vi "fitting modified.vi"(0 "fitting type":i8(ring), 5 "2D data":dbl[][](array[numeric]), 9 "force guess?":bool, 11 "intial guess value":dbl[](array[numeric])) -> (3 "number of function calls":i32 caption="函数调用次数", 6 "best fit":dbl[][](array[numeric]), 10 "best fit parameters":dbl[](array[numeric]))   [LabVIEW 2013]
uses:
  <vilib>/gmath/NumericalOptimization/Nonlinear Curve Fit LM.vi
  <vilib>/gmath/NI_Gmath.lvlib
panel:
  out "initial value 3":dbl[](array[numeric])
  out "sub3":dbl[][](array[numeric])
  out "split 2":dbl
  out "split 1":dbl
  in  "initial value 2":dbl[](array[numeric])
  in  "initial value 1":dbl[](array[numeric])
  in  "sub2":dbl[][](array[numeric])
  in  "sub1":dbl[][](array[numeric])
  in  "yc":dbl[](array[numeric])
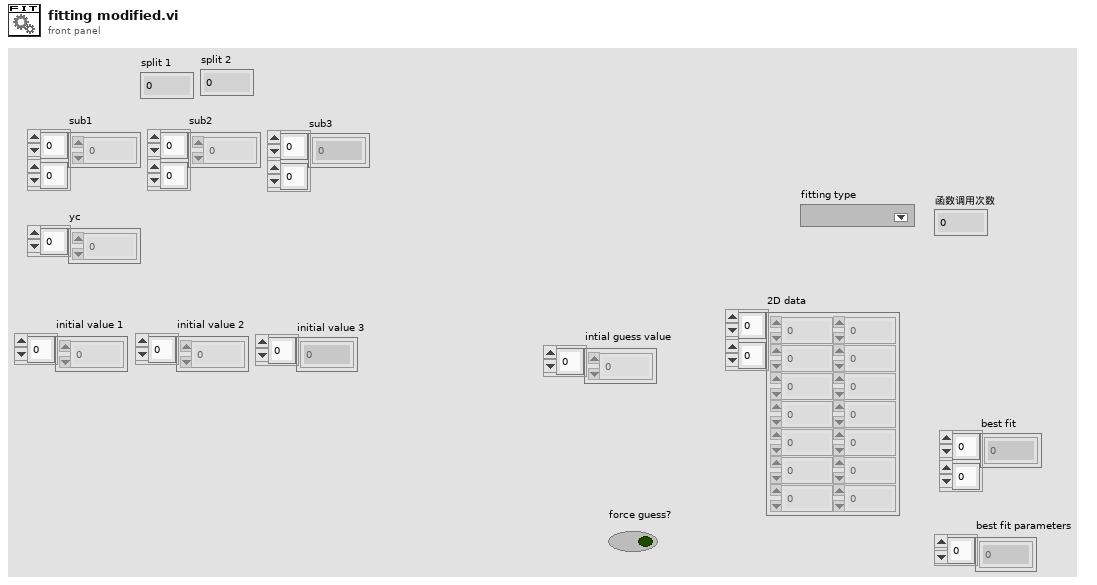
[diagram p1: front panel]
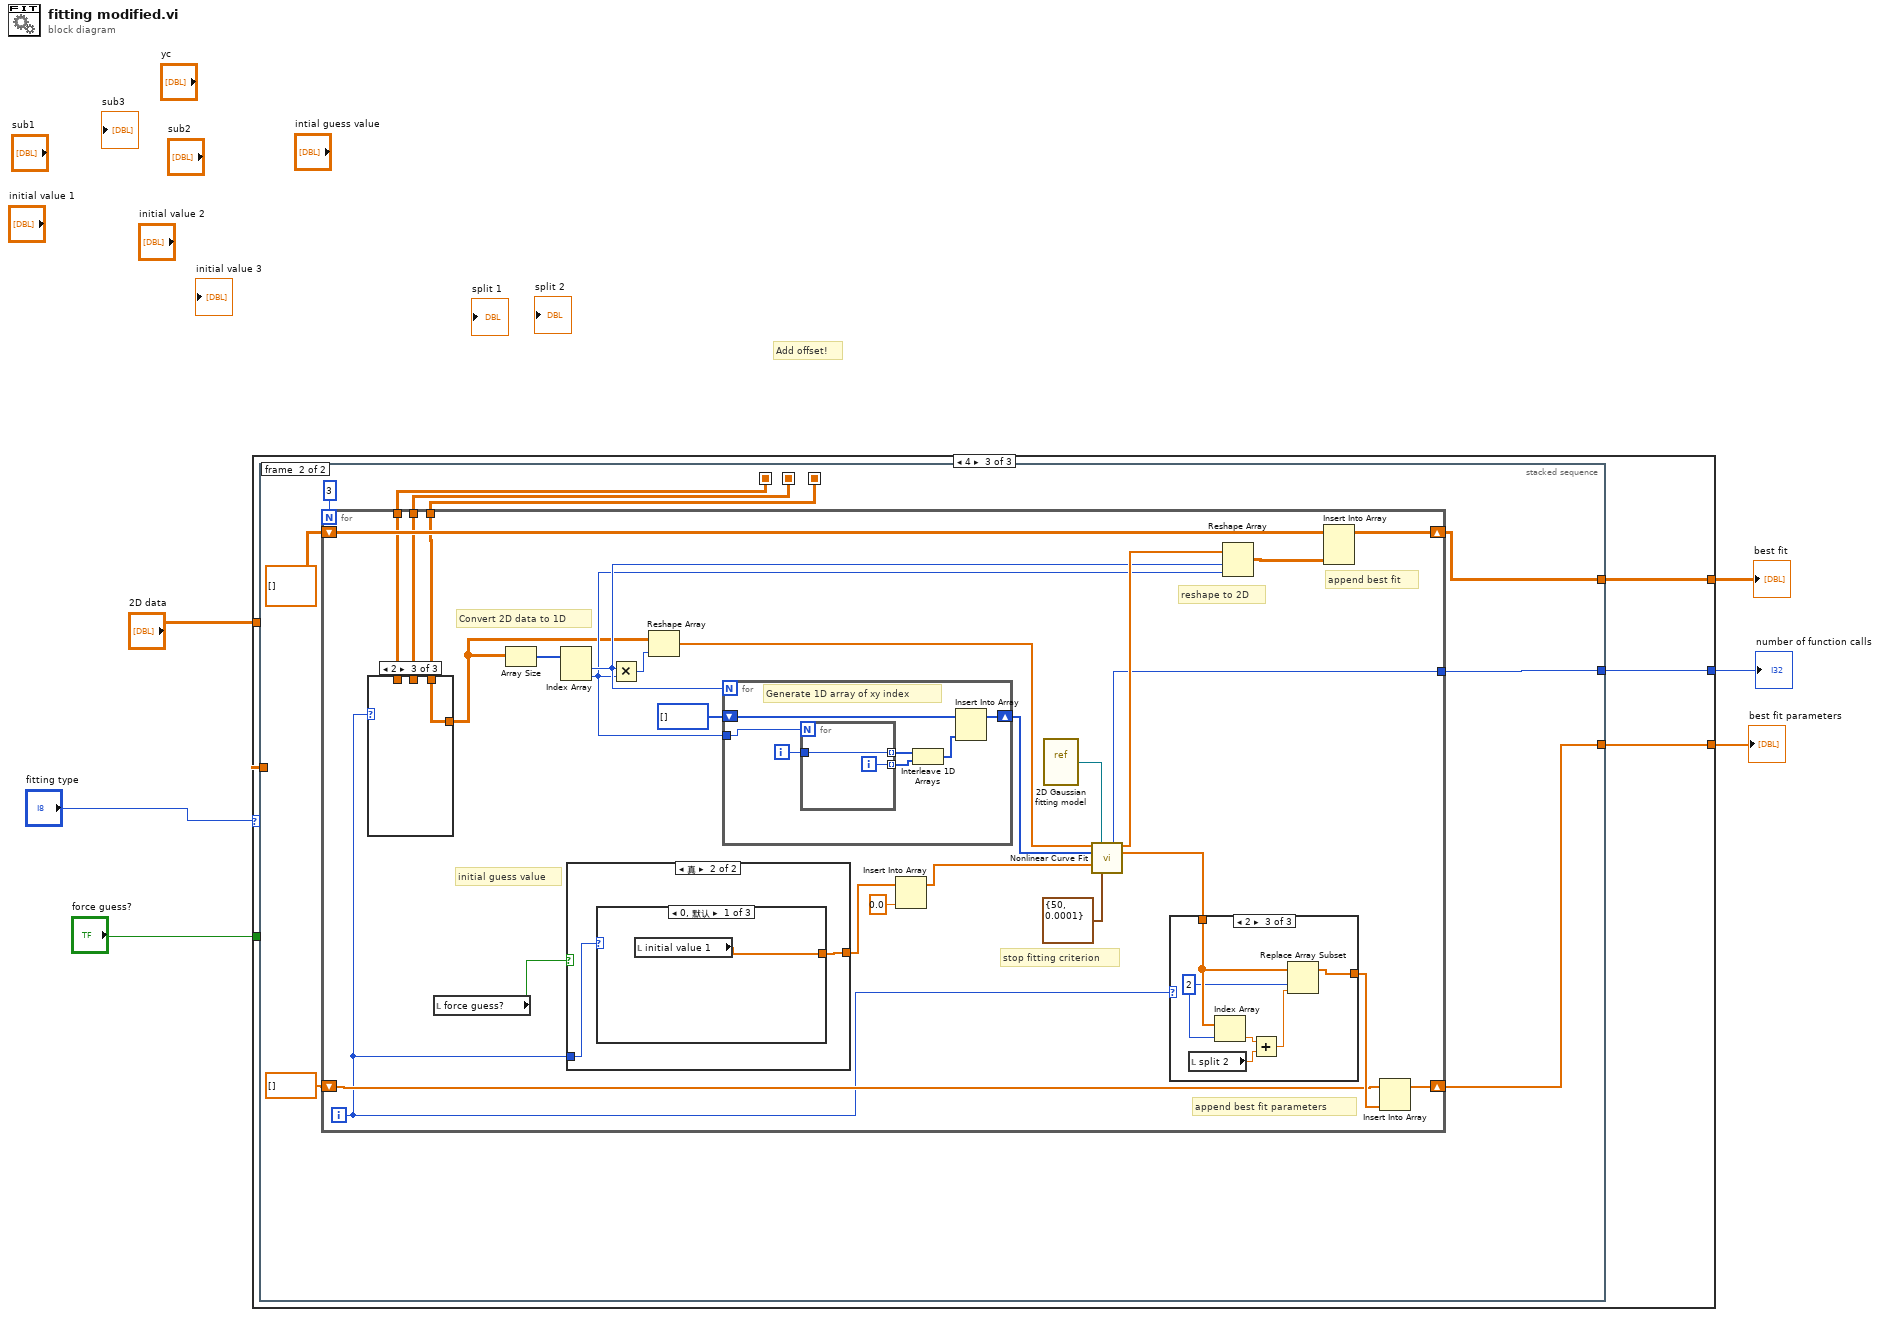
[diagram p0: block diagram]
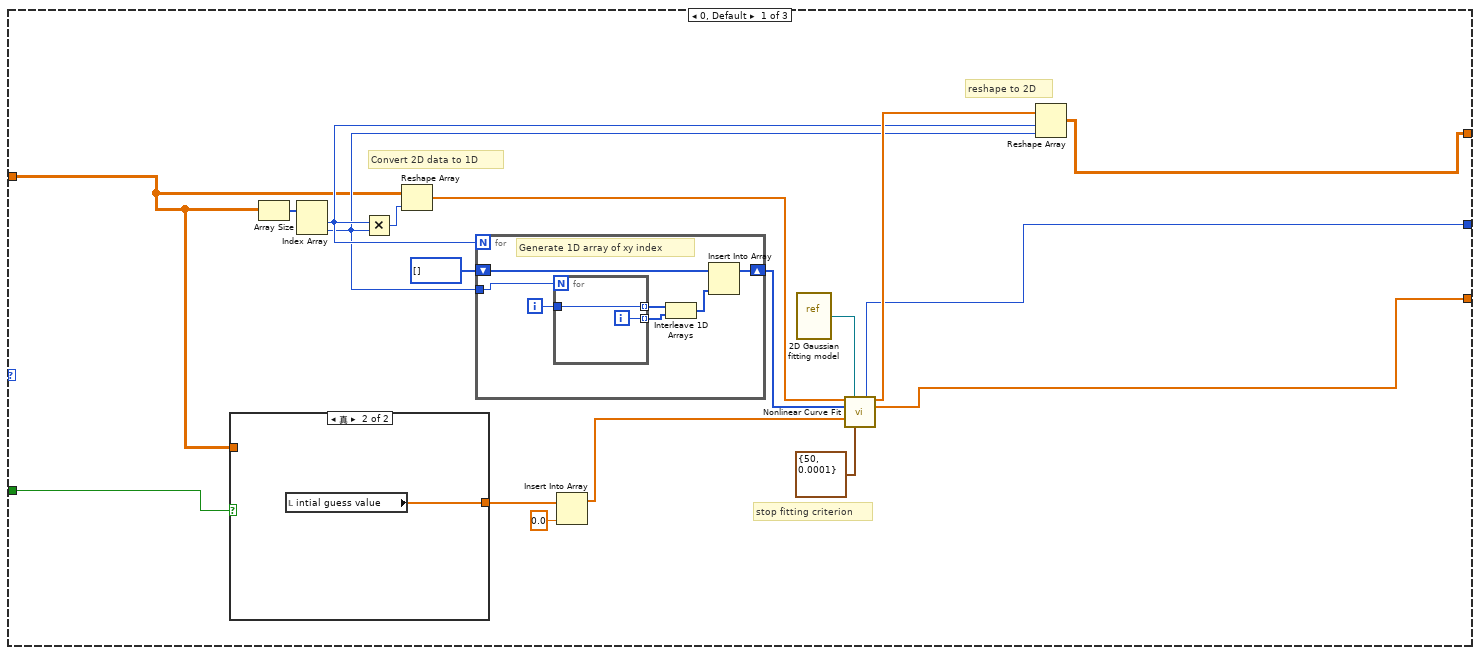
[diagram p2: hidden frame]
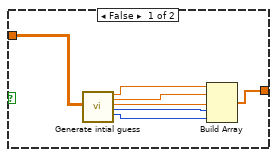
[diagram p3: hidden frame]
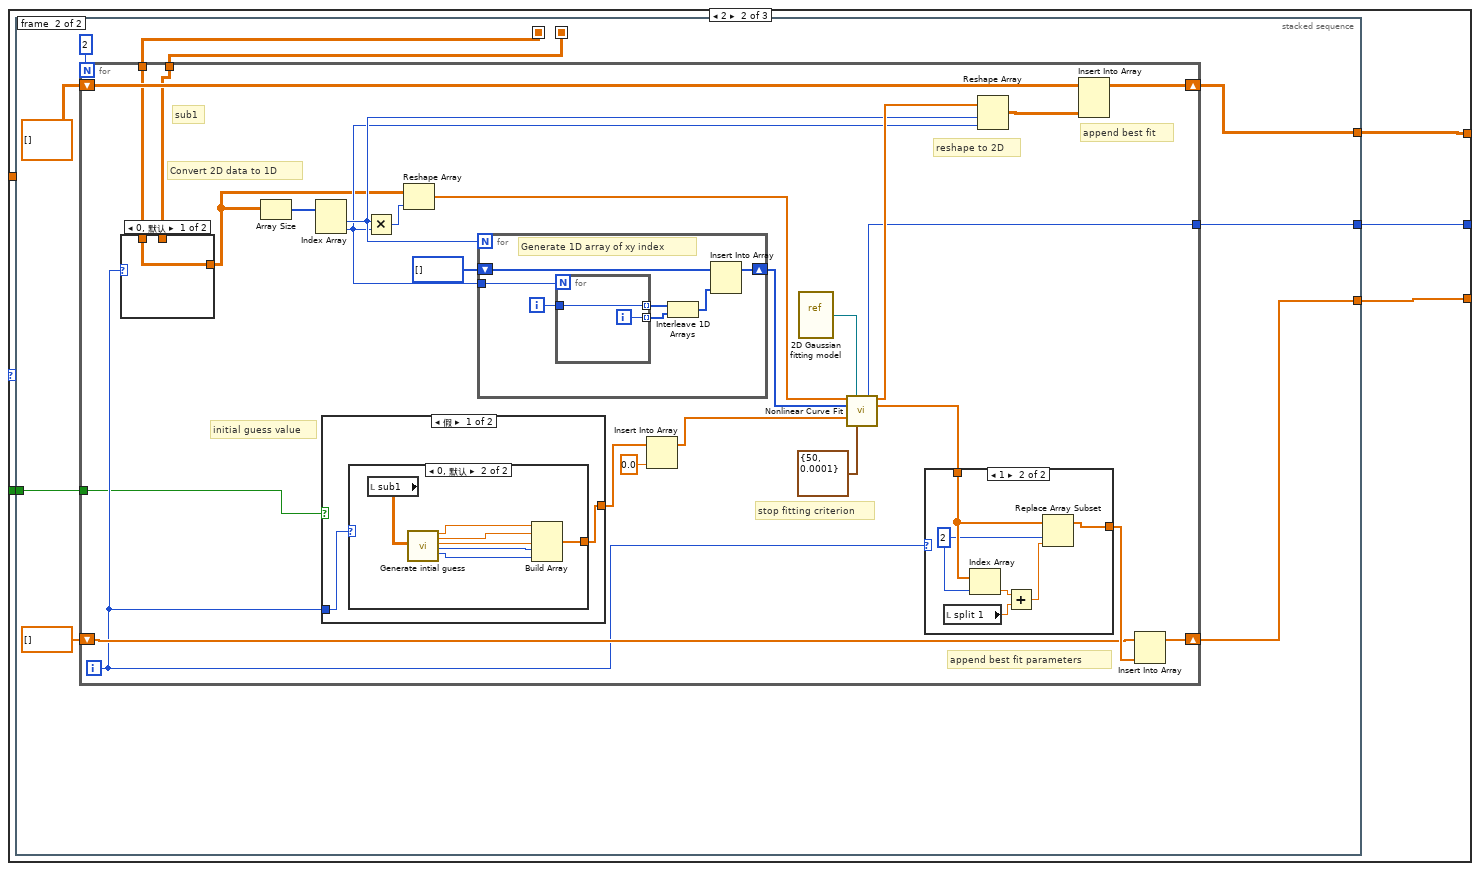
[diagram p4: hidden frame]
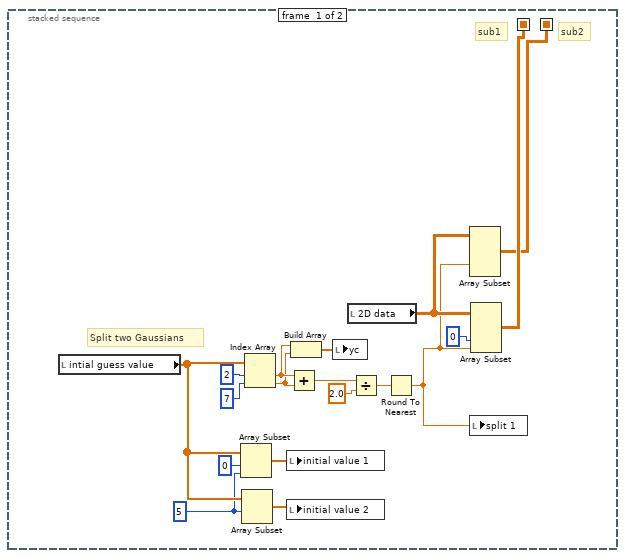
[diagram p5: hidden frame]
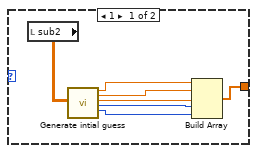
[diagram p8: hidden frame]
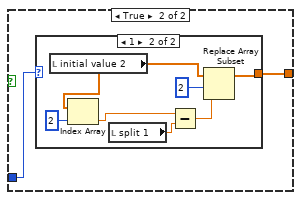
[diagram p9: hidden frame]
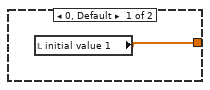
[diagram p10: hidden frame]
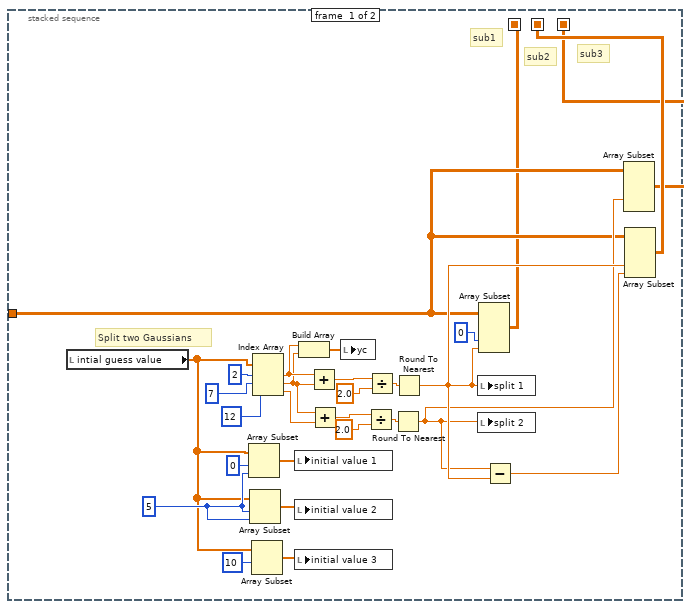
[diagram p11: hidden frame]
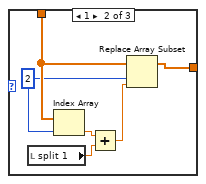
[diagram p15: hidden frame]
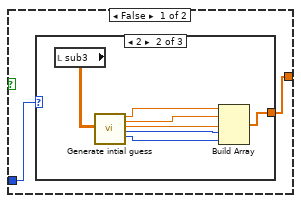
[diagram p16: hidden frame]
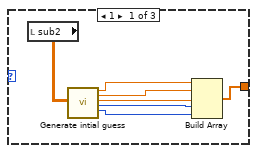
[diagram p17: hidden frame]
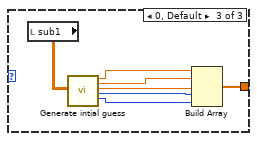
[diagram p18: hidden frame]
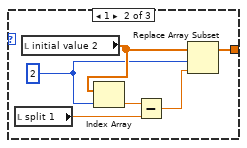
[diagram p19: hidden frame]
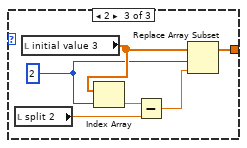
[diagram p20: hidden frame]
diagram:
  # "Add offset!"
  n1 = case shown="4" "fitting type" {
    tunnel: "2D data" -> [w11 _ w143]
    tunnel: [w14 w45 w146] -> w5
    tunnel: [w13 w44 w145] -> w4
    tunnel: [w12 w43 w144] -> w3
    tunnel: "force guess?" -> [w10 w42 _]
    frame 0, Default {
      # "Convert 2D data to 1D"
      # "reshape to 2D"
      # "stop fitting criterion"
      n2 = case shown="真" w10 {
        tunnel: [w35 w41] -> w9
        tunnel: w11 -> [w34 _]
        frame False {
          n3 = call "Generate intial guess.vi"("数组"=w34) -> ("peak"=w40:dbl, "xc"=w39:dbl, "yc"=w38:dbl, "sigx"=w37:i32, "sigy"=w36:i32)  [unwired: 14 in]
          n4 = Build Array(w40, w39, w38, w37, w36) -> (w35:dbl[])
        }
        frame True {
          n5 = local read "intial guess value"() -> (w41:dbl[])
        }
      }
      n6 = Array Size(array=w11) -> (size(s)=w21:i32[])
      n7 = Index Array(array=w21) -> (element #1=w17:i32, element #2=w16:i32)  [unwired: 2 in]
      n8 = Multiply(x=w17, y=w16) -> (x*y=w22:i32)
      n9 = Reshape Array(w11, w22) -> (w20:dbl[])
      n10 = for {
        N: w17 -> [_]
        shift-right: [w30] -> w15
        shift-left: i32[] [] -> [w29]
        tunnel: w16 -> [w25]
        i -> [w31]
        # "Generate 1D array of xy index"
        n11 = for {
          N: w25 -> [_]
          tunnel: [w33] -> w27 mode=indexing
          tunnel: w31 -> [w33]
          tunnel: [w32] -> w26 mode=indexing
          i -> [w32]
        }
        n12 = Interleave 1D Arrays(w27, w26) -> (w28:i32[])
        n13 = Insert Into Array(array=w29, new element=w28) -> (w30:i32[])  [unwired: 1 in]
      }
      n14 = Insert Into Array(array=w9, new element=0.0 ("新元素/子数组")) -> (w7:dbl[])  [unwired: 1 in]
      n15 = vi-ref "2D Gaussian fitting model.vi"() -> (w18:refnum<vi>)
      n16 = call-poly <vilib>:"Nonlinear Curve Fit.vi"("Y"=w20, "f(x,a)"=w18, "X"=w15, "initial parameters"=w7, "termination"=cluster{"max iteration":i32, "tolerance":dbl} {"max iteration"=50, "tolerance"=0.0001}) -> ("number of function calls"=w13:i32, "best nonlinear fit"=w24:dbl[], "best fit parameters"=w12:dbl[])  [unwired: 5 in, 3 out]
      n17 = Reshape Array(w24, w17, w16) -> (w14:dbl[][])
    }
    frame 2 {
      n18 = stacked-sequence {
        seq-local: [w47 _] -> [_ w66]
        seq-local: [w46 _] -> [_ w65]
        tunnel: [_ w69] -> w45
        tunnel: [_ w68] -> w44
        tunnel: [_ w67] -> w43
        tunnel: w42 -> [_ w64]
        frame #0 {
          w51 = 5 ("索引")
          # "sub2"
          # "sub1"
          # "Split two Gaussians"
          n19 = local read "intial guess value"() -> (w53:dbl[])
          n20 = Array Subset(array=w53, index=0 ("索引"), length=w51) -> (w50:dbl[])
          n21 = Array Subset(array=w53, index=w51) -> (w49:dbl[])  [unwired: 1 in]
          n22 = Index Array(array=w53, index #1=2 ("索引"), index #2=7 ("索引")) -> (element #1=w56:dbl, element #2=w55:dbl)
          n23 = local write "initial value 1"(w50) -> ()
          n24 = local write "initial value 2"(w49) -> ()
          n25 = Add(x=w56, y=w55) -> (x+y=w59:dbl)
          n26 = Build Array(w56, w55) -> (w61:dbl[])
          n27 = local write "yc"(w61) -> ()
          n28 = local read "2D data"() -> (w54:dbl[][])
          n29 = Divide(x=w59, y=2.0) -> (x/y=w57:dbl)
          n30 = Round To Nearest(number=w57) -> (nearest integer value=w48:dbl)
          n31 = Array Subset(array=w54, index (col)=w48) -> (w46:dbl[][])  [unwired: 3 in]
          n32 = local write "split 1"(w48) -> ()
          n33 = Array Subset(array=w54, index (col)=0 ("索引"), length (col)=w48) -> (w47:dbl[][])  [unwired: 2 in]
        }
        frame #1 {
          n34 = for {
            N: 2 -> [_]
            shift-right: [w90] -> w69
            shift-left: dbl[][] [] -> [w89]
            shift-right: [w85] -> w67
            shift-left: dbl[] [] -> [w84]
            tunnel: [w79] -> w68
            tunnel: w66 -> [w77]
            tunnel: w65 -> [w78]
            tunnel: w64 -> [w76]
            i -> [w81]
            # "sub1"
            # "append best fit parameters"
            # "append best fit"
            # "initial guess value"
            # "Convert 2D data to 1D"
            # "reshape to 2D"
            # "stop fitting criterion"
            n35 = case shown="0, 默认" w81 {
              tunnel: [w99 w100] -> w80
              tunnel: w78 -> [_ w100]
              tunnel: w77 -> [w99 _]
              frame 0, Default {
              }
              frame 1 {
              }
            }
            n36 = Array Size(array=w80) -> (size(s)=w95:i32[])
            n37 = Index Array(array=w95) -> (element #1=w83:i32, element #2=w82:i32)  [unwired: 2 in]
            n38 = case shown="假" w76 {
              tunnel: [w118 w134] -> w75
              tunnel: w81 -> [w117 w133]
              frame False {
                n39 = case shown="0, 默认" w117 {
                  tunnel: [w120 w127] -> w118
                  frame 1 {
                    n40 = local read "sub2"() -> (w119:dbl[][])
                    n41 = call "Generate intial guess.vi"("数组"=w119) -> ("peak"=w125:dbl, "xc"=w124:dbl, "yc"=w123:dbl, "sigx"=w122:i32, "sigy"=w121:i32)  [unwired: 14 in]
                    n42 = Build Array(w125, w124, w123, w122, w121) -> (w120:dbl[])
                  }
                  frame 0, Default {
                    n43 = local read "sub1"() -> (w126:dbl[][])
                    n44 = call "Generate intial guess.vi"("数组"=w126) -> ("peak"=w132:dbl, "xc"=w131:dbl, "yc"=w130:dbl, "sigx"=w129:i32, "sigy"=w128:i32)  [unwired: 14 in]
                    n45 = Build Array(w132, w131, w130, w129, w128) -> (w127:dbl[])
                  }
                }
              }
              frame True {
                n46 = case shown="1" w133 {
                  tunnel: [w135 w136] -> w134
                  frame 0, Default {
                    n47 = local read "initial value 1"() -> (w135:dbl[])
                  }
                  frame 1 {
                    n48 = local read "initial value 2"() -> (w137:dbl[])
                    n49 = Index Array(array=w137, index=2 ("索引")) -> (element=w141:dbl)
                    n50 = local read "split 1"() -> (w140:dbl)
                    n51 = Subtract(x=w141, y=w140) -> (x-y=w138:dbl)
                    n52 = Replace Array Subset(array=w137, new element=w138, index=2 ("索引")) -> (w136:dbl[])
                  }
                }
              }
            }
            n53 = Multiply(x=w83, y=w82) -> (x*y=w96:i32)
            n54 = Reshape Array(w80, w96) -> (w94:dbl[])
            n55 = for {
              N: w83 -> [_]
              shift-right: [w113] -> w91
              shift-left: i32[] [] -> [w112]
              tunnel: w82 -> [w108]
              i -> [w114]
              # "Generate 1D array of xy index"
              n56 = for {
                N: w108 -> [_]
                tunnel: [w116] -> w110 mode=indexing
                tunnel: w114 -> [w116]
                tunnel: [w115] -> w109 mode=indexing
                i -> [w115]
              }
              n57 = Interleave 1D Arrays(w110, w109) -> (w111:i32[])
              n58 = Insert Into Array(array=w112, new element=w111) -> (w113:i32[])  [unwired: 1 in]
            }
            n59 = Insert Into Array(array=w75, new element=0.0 ("新元素/子数组")) -> (w73:dbl[])  [unwired: 1 in]
            n60 = vi-ref "2D Gaussian fitting model.vi"() -> (w92:refnum<vi>)
            n61 = call-poly <vilib>:"Nonlinear Curve Fit.vi"("Y"=w94, "f(x,a)"=w92, "X"=w91, "initial parameters"=w73, "termination"=cluster{"max iteration":i32, "tolerance":dbl} {"max iteration"=50, "tolerance"=0.0001}) -> ("number of function calls"=w79:i32, "best nonlinear fit"=w98:dbl[], "best fit parameters"=w87:dbl[])  [unwired: 5 in, 3 out]
            n62 = case shown="1" w81 {
              tunnel: w87 -> [w101 w107]
              tunnel: [w101 w102] -> w86
              frame 0, Default {
              }
              frame 1 {
                w106 = 2 ("索引")
                n63 = local read "split 1"() -> (w104:dbl)
                n64 = Index Array(array=w107, index=w106) -> (element=w105:dbl)
                n65 = Add(x=w105, y=w104) -> (x+y=w103:dbl)
                n66 = Replace Array Subset(array=w107, new element=w103, index=w106) -> (w102:dbl[])
              }
            }
            n67 = Reshape Array(w98, w83, w82) -> (w88:dbl[][])
            n68 = Insert Into Array(array=w89, new element=w88) -> (w90:dbl[][])  [unwired: 2 in]
            n69 = Insert Into Array(array=w84, new element=w86) -> (w85:dbl[])  [unwired: 1 in]
          }
        }
      }
    }
    frame 4 {
      n70 = stacked-sequence {
        seq-local: [w149 _] -> [_ w177]
        seq-local: [w148 _] -> [_ w176]
        seq-local: [w147 _] -> [_ w175]
        tunnel: [_ w180] -> w146
        tunnel: [_ w179] -> w145
        tunnel: [_ w178] -> w144
        tunnel: w143 -> [w150 _]
        frame #0 {
          w154 = 5 ("索引")
          # "sub3"
          # "sub2"
          # "sub1"
          # "Split two Gaussians"
          n71 = local read "intial guess value"() -> (w153:dbl[])
          n72 = Array Subset(array=w153, index=0 ("索引"), length=w154) -> (w165:dbl[])
          n73 = Array Subset(array=w153, index=w154, length=w154) -> (w164:dbl[])
          n74 = Array Subset(array=w153, index=10 ("索引")) -> (w151:dbl[])  [unwired: 1 in]
          n75 = Index Array(array=w153, index #1=2 ("索引"), index #2=7 ("索引"), index #3=12 ("索引")) -> (element #1=w167:dbl, element #2=w159:dbl, element #3=w158:dbl)
          n76 = local write "initial value 1"(w165) -> ()
          n77 = local write "initial value 2"(w164) -> ()
          n78 = local write "initial value 3"(w151) -> ()
          n79 = Build Array(w167, w159) -> (w172:dbl[])
          n80 = Add(x=w167, y=w159) -> (x+y=w170:dbl)
          n81 = Add(x=w159, y=w158) -> (x+y=w162:dbl)
          n82 = local write "yc"(w172) -> ()
          n83 = Divide(x=w162, y=2.0) -> (x/y=w160:dbl)
          n84 = Divide(x=w170, y=2.0) -> (x/y=w168:dbl)
          n85 = Round To Nearest(number=w160) -> (nearest integer value=w155:dbl)
          n86 = Round To Nearest(number=w168) -> (nearest integer value=w157:dbl)
          n87 = local write "split 1"(w157) -> ()
          n88 = local write "split 2"(w155) -> ()
          n89 = Array Subset(array=w150, index (col)=0 ("索引"), length (col)=w157) -> (w149:dbl[][])  [unwired: 2 in]
          n90 = Subtract(x=w155, y=w157) -> (x-y=w156:dbl)
          n91 = Array Subset(array=w150, index (col)=w155) -> (w147:dbl[][])  [unwired: 3 in]
          n92 = Array Subset(array=w150, index (col)=w157, length (col)=w156) -> (w148:dbl[][])  [unwired: 2 in]
        }
        frame #1 {
          n93 = for {
            N: 3 -> [_]
            shift-right: [w201] -> w180
            shift-left: dbl[][] [] -> [w200]
            shift-right: [w196] -> w178
            shift-left: dbl[] [] -> [w195]
            tunnel: [w190] -> w179
            tunnel: w177 -> [w189]
            tunnel: w176 -> [w188]
            tunnel: w175 -> [w187]
            i -> [w192]
            # "append best fit parameters"
            # "append best fit"
            # "initial guess value"
            # "Convert 2D data to 1D"
            # "reshape to 2D"
            # "stop fitting criterion"
            n94 = case shown="2" w192 {
              tunnel: [w211 w212 w213] -> w191
              tunnel: w189 -> [w211 _ _]
              tunnel: w188 -> [_ w212 _]
              tunnel: w187 -> [_ _ w213]
              frame 0, Default {
              }
              frame 1 {
              }
              frame 2 {
              }
            }
            n95 = local read "force guess?"() -> (w208:bool)
            n96 = Array Size(array=w191) -> (size(s)=w206:i32[])
            n97 = Index Array(array=w206) -> (element #1=w194:i32, element #2=w193:i32)  [unwired: 2 in]
            n98 = case shown="真" w208 {
              tunnel: [w237 w260] -> w186
              tunnel: w192 -> [w236 w259]
              frame False {
                n99 = case shown="2" w236 {
                  tunnel: [w239 w246 w253] -> w237
                  frame 1 {
                    n100 = local read "sub2"() -> (w238:dbl[][])
                    n101 = call "Generate intial guess.vi"("数组"=w238) -> ("peak"=w244:dbl, "xc"=w243:dbl, "yc"=w242:dbl, "sigx"=w241:i32, "sigy"=w240:i32)  [unwired: 14 in]
                    n102 = Build Array(w244, w243, w242, w241, w240) -> (w239:dbl[])
                  }
                  frame 2 {
                    n103 = local read "sub3"() -> (w245:dbl[][])
                    n104 = call "Generate intial guess.vi"("数组"=w245) -> ("peak"=w251:dbl, "xc"=w250:dbl, "yc"=w249:dbl, "sigx"=w248:i32, "sigy"=w247:i32)  [unwired: 14 in]
                    n105 = Build Array(w251, w250, w249, w248, w247) -> (w246:dbl[])
                  }
                  frame 0, Default {
                    n106 = local read "sub1"() -> (w252:dbl[][])
                    n107 = call "Generate intial guess.vi"("数组"=w252) -> ("peak"=w258:dbl, "xc"=w257:dbl, "yc"=w256:dbl, "sigx"=w255:i32, "sigy"=w254:i32)  [unwired: 14 in]
                    n108 = Build Array(w258, w257, w256, w255, w254) -> (w253:dbl[])
                  }
                }
              }
              frame True {
                n109 = case shown="0, 默认" w259 {
                  tunnel: [w261 w262 w268] -> w260
                  frame 0, Default {
                    n110 = local read "initial value 1"() -> (w261:dbl[])
                  }
                  frame 1 {
                    w264 = 2 ("索引")
                    n111 = local read "split 1"() -> (w266:dbl)
                    n112 = local read "initial value 2"() -> (w265:dbl[])
                    n113 = Index Array(array=w265, index=w264) -> (element=w267:dbl)
                    n114 = Subtract(x=w267, y=w266) -> (x-y=w263:dbl)
                    n115 = Replace Array Subset(array=w265, new element=w263, index=w264) -> (w262:dbl[])
                  }
                  frame 2 {
                    w270 = 2 ("索引")
                    n116 = local read "split 2"() -> (w272:dbl)
                    n117 = local read "initial value 3"() -> (w271:dbl[])
                    n118 = Index Array(array=w271, index=w270) -> (element=w273:dbl)
                    n119 = Subtract(x=w273, y=w272) -> (x-y=w269:dbl)
                    n120 = Replace Array Subset(array=w271, new element=w269, index=w270) -> (w268:dbl[])
                  }
                }
              }
            }
            n121 = Multiply(x=w194, y=w193) -> (x*y=w207:i32)
            n122 = Reshape Array(w191, w207) -> (w205:dbl[])
            n123 = for {
              N: w194 -> [_]
              shift-right: [w232] -> w202
              shift-left: i32[] [] -> [w231]
              tunnel: w193 -> [w227]
              i -> [w233]
              # "Generate 1D array of xy index"
              n124 = for {
                N: w227 -> [_]
                tunnel: [w235] -> w229 mode=indexing
                tunnel: w233 -> [w235]
                tunnel: [w234] -> w228 mode=indexing
                i -> [w234]
              }
              n125 = Interleave 1D Arrays(w229, w228) -> (w230:i32[])
              n126 = Insert Into Array(array=w231, new element=w230) -> (w232:i32[])  [unwired: 1 in]
            }
            n127 = Insert Into Array(array=w186, new element=0.0 ("新元素/子数组")) -> (w184:dbl[])  [unwired: 1 in]
            n128 = vi-ref "2D Gaussian fitting model.vi"() -> (w203:refnum<vi>)
            n129 = call-poly <vilib>:"Nonlinear Curve Fit.vi"("Y"=w205, "f(x,a)"=w203, "X"=w202, "initial parameters"=w184, "termination"=cluster{"max iteration":i32, "tolerance":dbl} {"max iteration"=50, "tolerance"=0.0001}) -> ("number of function calls"=w190:i32, "best nonlinear fit"=w210:dbl[], "best fit parameters"=w198:dbl[])  [unwired: 5 in, 3 out]
            n130 = case shown="2" w192 {
              tunnel: w198 -> [w214 w220 w226]
              tunnel: [w214 w215 w221] -> w197
              frame 0, Default {
              }
              frame 1 {
                w219 = 2 ("索引")
                n131 = local read "split 1"() -> (w217:dbl)
                n132 = Index Array(array=w220, index=w219) -> (element=w218:dbl)
                n133 = Add(x=w218, y=w217) -> (x+y=w216:dbl)
                n134 = Replace Array Subset(array=w220, new element=w216, index=w219) -> (w215:dbl[])
              }
              frame 2 {
                w225 = 2 ("索引")
                n135 = local read "split 2"() -> (w223:dbl)
                n136 = Index Array(array=w226, index=w225) -> (element=w224:dbl)
                n137 = Add(x=w224, y=w223) -> (x+y=w222:dbl)
                n138 = Replace Array Subset(array=w226, new element=w222, index=w225) -> (w221:dbl[])
              }
            }
            n139 = Reshape Array(w210, w194, w193) -> (w199:dbl[][])
            n140 = Insert Into Array(array=w200, new element=w199) -> (w201:dbl[][])  [unwired: 2 in]
            n141 = Insert Into Array(array=w195, new element=w197) -> (w196:dbl[])  [unwired: 1 in]
          }
        }
      }
    }
  }
  "number of function calls" <- w4
  "best fit parameters" <- w3
  "best fit" <- w5
